vi "CLSUIP_ResizeBDWin.vi"(8 "error in (no error)":errorcluster, 11 "VI Refnum":refnum<vi>) -> (0 "error out":errorcluster, 3 "VI Refnum out":refnum<vi>)   [LabVIEW 2021, in "MemberVICreation.lvlib"]
uses:
  <resource>/Framework/Providers/LVClassLibrary/NewAccessors/MemberVICreation.lvlib
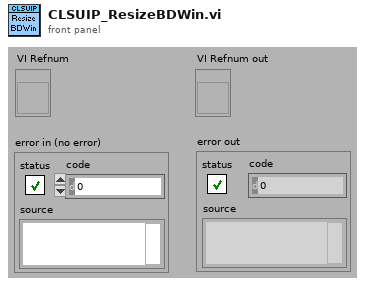
[diagram p1: front panel]
types:
  T1 = cluster{"left":i16, "top":i16, "right":i16, "bottom":i16}
  T2 = typedef "LVRectTypeDef.ctl" = cluster{"left":i16, "top":i16, "right":i16, "bottom":i16}
  T3 = typedef "LVBoundsTypeDef.ctl" = cluster{"Width":u32, "Height":u32}
  T4 = typedef "LVPointTypeDef.ctl" = cluster{"Horizontal":i16, "Vertical":i16}
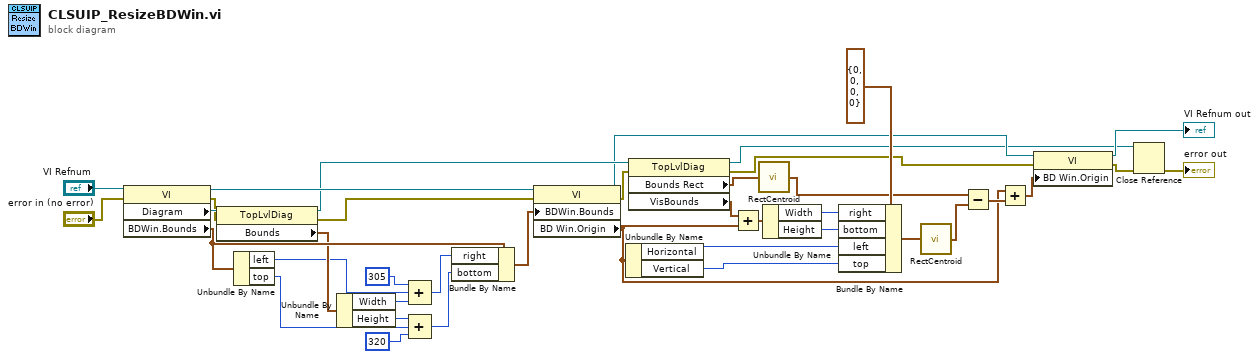
[diagram p0: block diagram]
diagram:
  n1 = property on="Property Node" class="VI"(reference="VI Refnum", error in="error in (no error)") -> (reference out=w35:refnum<vi>, error out=w36:errorcluster, "Diagram"=w37:refnum<vi>, "BDWin.Bounds"=w33:T2)
  n2 = property on="Property Node" class="TopLvlDiag"(reference=w37, error in=w36) -> (reference out=w20:refnum<vi>, error out=w34:errorcluster, "Bounds"=w32:T3)
  n3 = Unbundle By Name(w33) -> ("left"=w27:i16, "top"=w25:i16)
  n4 = Unbundle By Name(w32) -> ("Width"=w29:u32, "Height"=w28:u32)
  n5 = Compound Arithmetic op=ADD(i16 305 ("value"), w27, w29) -> (w23:u32)
  n6 = Compound Arithmetic op=ADD(w28, w25, i16 320 ("value")) -> (w22:u32)
  n7 = Bundle By Name(cluster=w33, "right"=w23, "bottom"=w22) -> (w31:T2)
  n8 = property on="Property Node" class="VI"(reference=w35, error in=w34, "BDWin.Bounds"=w31) -> (reference out=w7:refnum<vi>, error out=w21:errorcluster, "BD Win.Origin"=w1:T4)
  n9 = Unbundle By Name(w1) -> ("Horizontal"=w18:i16, "Vertical"=w17:i16)
  n10 = property on="Property Node" class="TopLvlDiag"(reference=w20, error in=w21) -> (reference out=w4:refnum<vi>, error out=w8:errorcluster, "Bounds Rect"=w11:T2, "VisBounds"=w16:T3)
  n11 = Add(x=w16, y=w1) -> (x+y=w14:T3)
  n12 = call <vilib>:"RectCentroid.vi"("rect"=w11) -> ("point"=w9:cluster{"x":i16, "y":i16})
  n13 = Unbundle By Name(w14) -> ("Width"=w15:u32, "Height"=w13:u32)
  n14 = Bundle By Name(cluster=T1 {"left"=0, "top"=0, "right"=0, "bottom"=0} ("rect"), "right"=w15, "bottom"=w13, "left"=w18, "top"=w17) -> (w12:T1)
  n15 = call <vilib>:"RectCentroid.vi"("rect"=w12) -> ("point"=w10:cluster{"x":i16, "y":i16})
  n16 = Subtract(x=w9, y=w10) -> (x-y=w2:cluster{"x":i16, "y":i16})
  n17 = Add(x=w1, y=w2) -> (x+y=w3:T4)
  n18 = property on="Property Node" class="VI"(reference=w7, error in=w8, "BD Win.Origin"=w3) -> (reference out=→"VI Refnum out":refnum<vi>, error out=w6:errorcluster)
  n19 = Close Reference(reference=w4, error in (no error)=w6) -> (error out=→"error out":errorcluster)
